vi "CreateFolder.vi"() -> (0 "Bool":bool, 2 "Return":string)   [LabVIEW 2017]
panel:
  in  "Msg":string="Input folder name."
  in  "Cancel 2":bool
  in  "OK 2":bool
  in  "ファイル名":string
  # "フォルダ名"
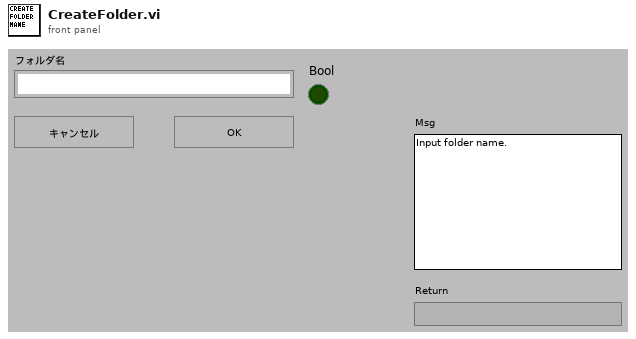
[diagram p1: front panel]
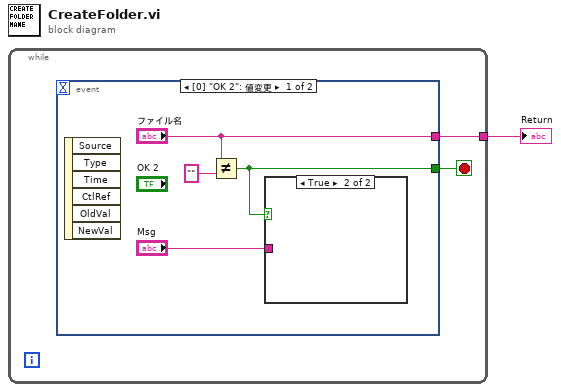
[diagram p0: block diagram]
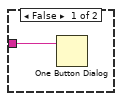
[diagram p2: hidden frame]
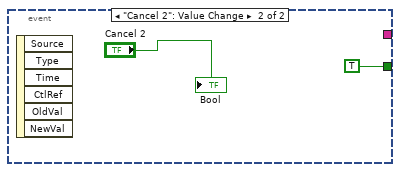
[diagram p3: hidden frame]
diagram:
  n1 = while {
    tunnel: [w2] -> w1
    stop <- w3 stop-if-true
    n2 = event shown="[0] \"OK 2\": 値変更" {
      selector: _ -> [_ _]
      dyn-events: _ -> [_ _]
      timeout: _ -> [_ _]
      tunnel: ["ファイル名" _] -> w2
      tunnel: [w5 TRUE] -> w3
      event "OK 2": Value Change {
        n3 = event-data() -> ()  [unwired: 1 in, 6 out]
        n4 = Not Equal?(x="ファイル名", y="") -> (x != y?=w5:bool)
        n5 = case shown="TRUE" w5 {
          tunnel: "Msg" -> [w8 _]
          frame False {
            n6 = One Button Dialog(message=w8) -> ()  [unwired: 1 in, 1 out]
          }
          frame True {
          }
        }
      }
      event "Cancel 2": Value Change {
        n7 = event-data() -> ()  [unwired: 1 in, 6 out]
        "Bool" <- "Cancel 2"
      }
    }
  }
  "Return" <- w1
